vi "Destroy Table Buffer.vi"(8 "error in":errorcluster) -> (0 "error out":errorcluster)   [LabVIEW 2025, in "Automotive Ethernet Bus Monitor UI.lvlib"]
doc: "Destroy the Table Buffer."
uses:
  Automotive Ethernet Bus Monitor UI.lvlib
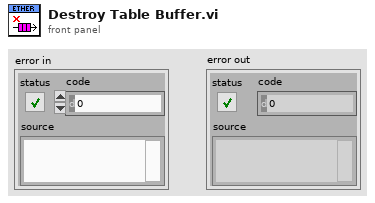
[diagram p1: front panel]
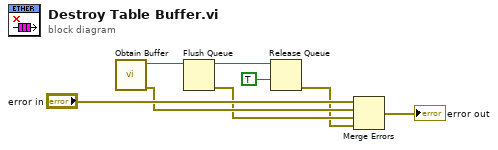
[diagram p0: block diagram]
diagram:
  n1 = call "Obtain Buffer.vi"() -> ("error out"=w4:errorcluster, "Table Queue"=w6:refnum<queue>)  [unwired: 10 in]
  n2 = Flush Queue(queue=w6) -> (queue out=w5:refnum<queue>, error out=w3:errorcluster)  [unwired: 1 in, 1 out]
  n3 = Release Queue(queue=w5, force destroy? (F)=TRUE) -> (error out=w2:errorcluster)  [unwired: 1 in, 2 out]
  n4 = Merge Errors("error in", w4, w3, w2) -> (→"error out":errorcluster)
